vi "Time lapse wait for next frame - subvi.vi"(8 "Error In":errorcluster, 10 "Frame Interval (s)":dbl format="%#_13g", 11 "Time of last frame in":u32) -> (0 "Error Out":errorcluster, 1 "Stopped?":bool, 2 "Sec. till next frame":ext(slide), 3 "Time of this frame out (ms)":i32)   [LabVIEW 2014]
uses:
  Shutter Control/Shutter SubVIs/ctts/control shutters.ctl
  Shutter Control/Shutter SubVIs/Global Shutter Variables - SubVI.vi
  TIRF Lock/autofocus-globals.vi
panel:
  in  "stop":bool
  in  "GO NOW!":bool
  in  "Pause":bool
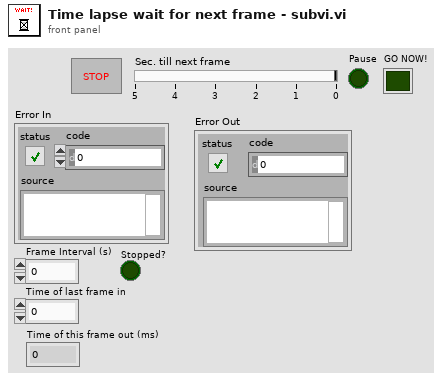
[diagram p1: front panel]
types:
  T1 = typedef "control shutters.ctl" = cluster{"Camera Shutter":bool, "Laser Shutter":enum32{"No Selection", "GFP", "Cy3 Long \nPass", "Cy3", "Cy5", "Off"}}
  T2 = typedef "laser shutters.ctl" = enum32{"No Selection", "GFP", "Cy3 Long \nPass", "Cy3", "Cy5", "Off", "IR"}
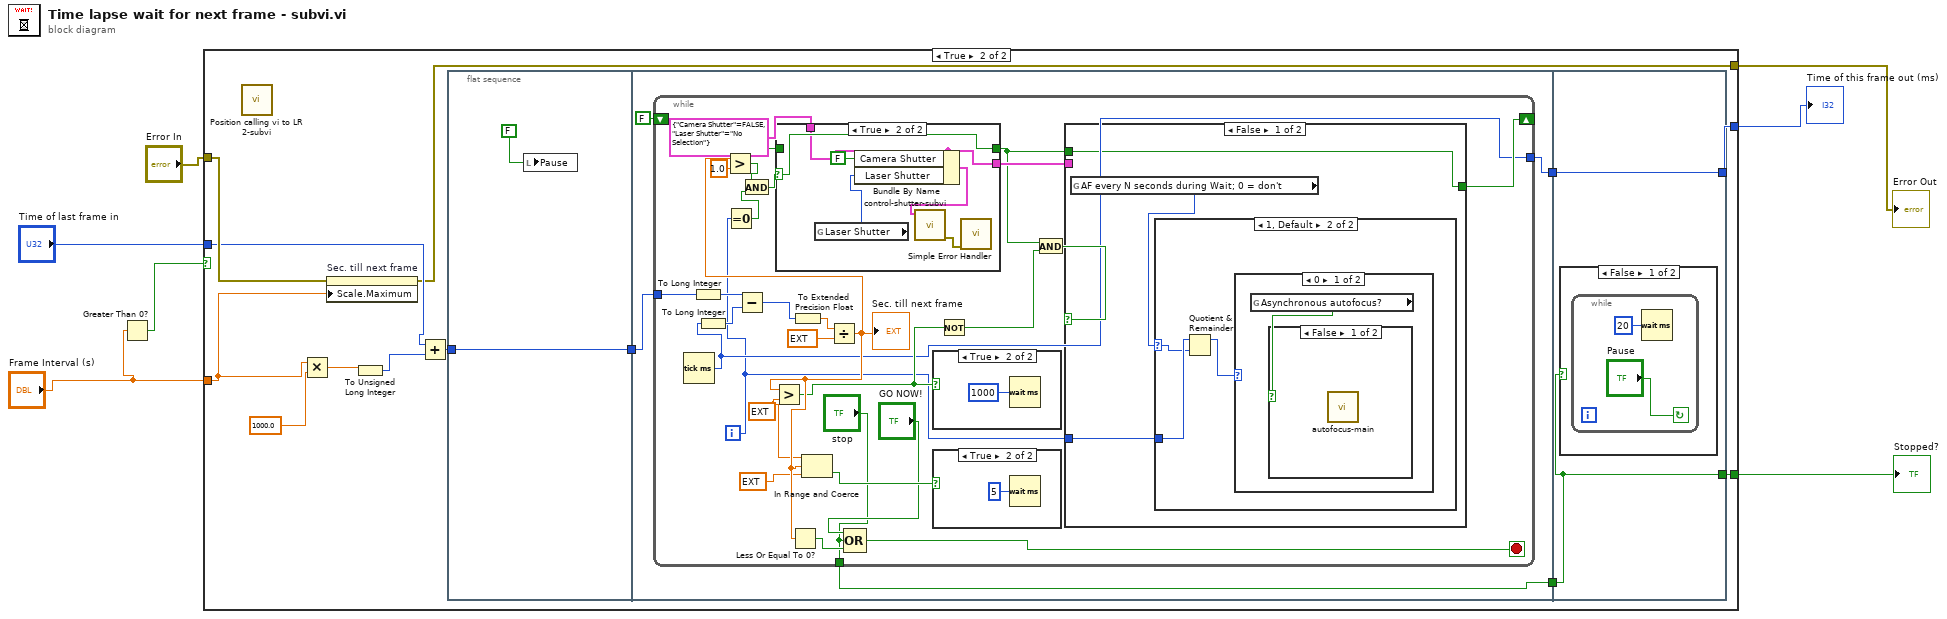
[diagram p0: block diagram]
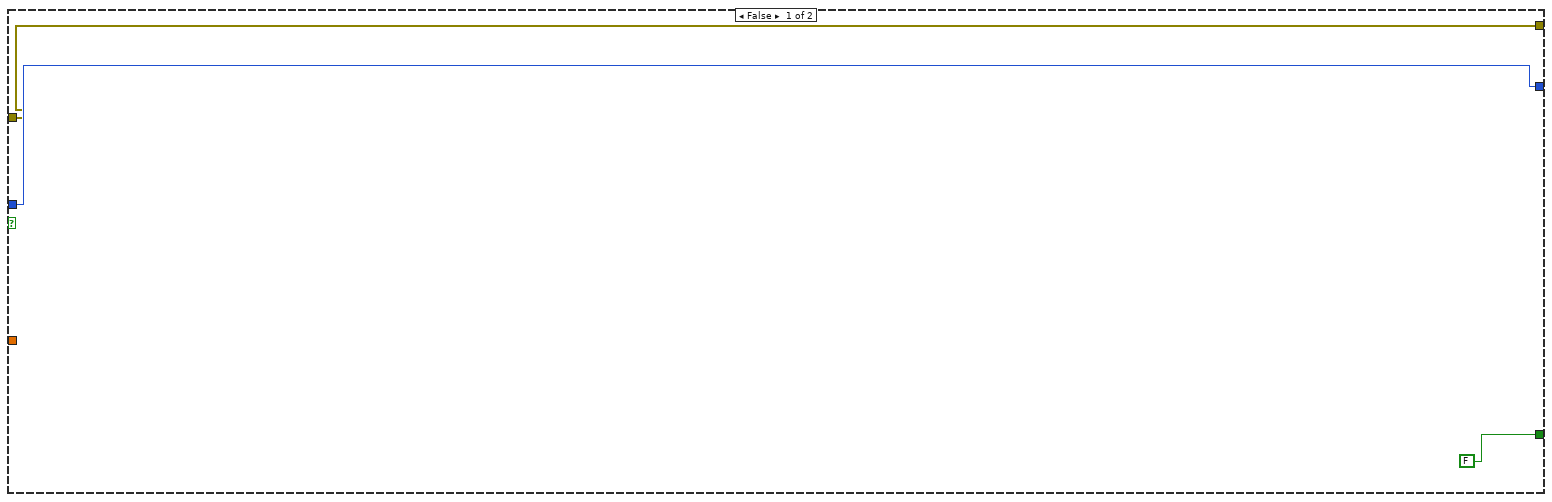
[diagram p2: hidden frame]
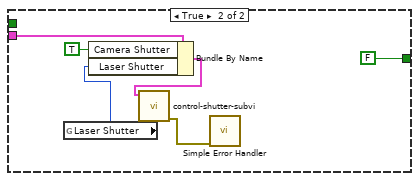
[diagram p6: hidden frame]
diagram:
  n1 = Greater Than 0?(x="Frame Interval (s)") -> (x > 0?=w4:bool)
  n2 = case shown="True" w4 {
    tunnel: "Error In" -> [w8 w23]
    tunnel: "Time of last frame in" -> [w10 w18]
    tunnel: "Frame Interval (s)" -> [_ w22]
    tunnel: [w10 w13] -> w3
    tunnel: [FALSE w14] -> w2
    tunnel: [w8 w11] -> w1
    frame False {
    }
    frame True {
      n3 = call "Position calling vi to LR 2-subvi.vi"() -> ()  [unwired: 4 in, 2 out]
      n4 = Multiply(x=w22, y=1000.0) -> (x*y=w20:dbl)
      n5 = property on="Sec. till next frame" class="Slide (strict)"(error in=w23, "Scale.Maximum"=w22) -> (error out=w11:errorcluster)  [unwired: 1 in, 1 out]
      n6 = To Unsigned Long Integer(number=w20) -> (unsigned 32bit integer=w19:u32)
      n7 = Add(x=w18, y=w19) -> (x+y=w16:u32)
      n8 = flat-sequence {
        tunnel: [w24] -> w17
        tunnel: w16 -> [w24]
        tunnel: w17 -> [w28]
        tunnel: [w27] -> w15
        tunnel: [w26] -> w12
        tunnel: w15 -> [w82]
        tunnel: [w82] -> w14
        tunnel: [w81] -> w13
        tunnel: w12 -> [w81]
        frame #0 {
          n9 = local write "Pause"(FALSE) -> ()
        }
        frame #1 {
          n10 = while {
            shift-right: [w33] -> _
            shift-left: FALSE -> [w57]
            tunnel: w28 -> [w49]
            tunnel: ["stop"] -> w27
            tunnel: [w32] -> w26
            i -> [w31]
            stop <- w41 stop-if-true
            w45 = ext 1.04999999999999999996 ("y")
            n11 = Tick Count (ms)() -> (millisecond timer value=w32:u32)
            n12 = To Long Integer(number=w49) -> (32bit integer=w52:i32)
            n13 = To Long Integer(number=w32) -> (32bit integer=w51:i32)
            n14 = Equal To 0?(x=w31) -> (x = 0?=w54:bool)
            n15 = Subtract(x=w52, y=w51) -> (x-y=w50:i32)
            n16 = To Extended Precision Float(1:w50) -> (0:w48:ext)
            n17 = Divide(x=w48, y=ext 1000.0) -> (x/y=w46:ext)
            "Sec. till next frame" <- w46
            n18 = Greater?(x=w46, y=1.0) -> (0:w55:bool)
            n19 = And(x=w55, y=w54) -> (x .and. y?=w56:bool)
            n20 = Greater?(x=w46, y=w45) -> (0:w37:bool)
            n21 = case shown="True" w56 {
              selector: w56 -> [_ w76]
              tunnel: w57 -> [w74 _]
              tunnel: [w74 w76] -> w30
              tunnel: [w73 w75] -> w35
              tunnel: T1 {"Camera Shutter"=FALSE, "Laser Shutter"=enum."No Selection"} ("Shutter Control") -> [w73 w75]
              frame False {
              }
              frame True {
                n22 = global read "Global Shutter Variables - SubVI.vi" "Laser Shutter"() -> (w78:T2)
                n23 = Bundle By Name(cluster=w75, "Camera Shutter"=FALSE, "Laser Shutter"=w78) -> (w80:T1)
                n24 = call "control-shutter-subvi.vi"("Shutter Control"=w80) -> ("Error Out"=w79:errorcluster)  [unwired: 10 in]
                n25 = call <vilib>:"Simple Error Handler.vi"("error in (no error)"=w79) -> ()  [unwired: 4 in, 5 out]
              }
            }
            n26 = Less Or Equal To 0?(x=w46) -> (x <= 0?=w42:bool)
            n27 = In Range and Coerce(upper limit=w45, x=w46, lower limit=ext 0.01 ("x/y")) -> (In Range?=w43:bool)  [unwired: 1 out]
            n28 = Compound Arithmetic op=OR("GO NOW!", "stop", w42) -> (w41:bool)
            n29 = case shown="True" w37 {
              frame False {
              }
              frame True {
                n30 = Wait (ms)(milliseconds to wait=u32 1000) -> ()  [unwired: 1 out]
              }
            }
            n31 = case shown="True" w43 {
              frame False {
              }
              frame True {
                n32 = Wait (ms)(milliseconds to wait=u32 5) -> ()  [unwired: 1 out]
              }
            }
            n33 = Not(x=w37) -> (.not. x?=w38:bool)
            n34 = And(x=w30, y=w38) -> (x .and. y?=w36:bool)
            n35 = case shown="False" w36 {
              tunnel: w35 -> [_ w70]
              tunnel: [w58 FALSE] -> w33
              tunnel: w31 -> [w59 _]
              tunnel: w30 -> [w58 _]
              frame False {
                n36 = global read "autofocus-globals.vi" "AF every N seconds during Wait; 0 = don't"() -> (w60:u32)
                n37 = case shown="1, Default" w60 {
                  selector: w60 -> [_ w62]
                  tunnel: w59 -> [_ w63]
                  frame 0 {
                  }
                  frame 1, Default {
                    n38 = Quotient & Remainder(x=w63, y=w62) -> (x-y*floor(x/y)=w61:u32)  [unwired: 1 out]
                    n39 = case shown="0" w61 {
                      frame 0 {
                        n40 = global read "autofocus-globals.vi" "Asynchronous autofocus?"() -> (w64:bool)
                        n41 = case shown="False" w64 {
                          frame False {
                            n42 = call "autofocus-main.vi"() -> ()  [unwired: 12 in]
                          }
                          frame True {
                          }
                        }
                      }
                      frame 1, Default {
                      }
                    }
                  }
                }
              }
              frame True {
                n43 = global read "Global Shutter Variables - SubVI.vi" "Laser Shutter"() -> (w68:T2)
                n44 = Bundle By Name(cluster=w70, "Camera Shutter"=TRUE, "Laser Shutter"=w68) -> (w67:T1)
                n45 = call "control-shutter-subvi.vi"("Shutter Control"=w67) -> ("Error Out"=w66:errorcluster)  [unwired: 10 in]
                n46 = call <vilib>:"Simple Error Handler.vi"("error in (no error)"=w66) -> ()  [unwired: 4 in, 5 out]
              }
            }
          }
        }
        frame #2 {
          n47 = case shown="False" w82 {
            frame False {
              n48 = while {
                stop <- "Pause" continue-if-true
                n49 = Wait (ms)(milliseconds to wait=u32 20) -> ()  [unwired: 1 out]
              }
            }
            frame True {
            }
          }
        }
      }
    }
  }
  "Error Out" <- w1
  "Stopped?" <- w2
  "Time of this frame out (ms)" <- w3
